vi "Man_Power Booking.vi"(6 "Man Power Details":T1={"Man Power"={"OP10"={"Clock No."="", "Name"=""}, "OP20"={"Clock No."="", "Name"=""}, "OP30"={"Clock No."="", "Name"=""}, "OP40"={"Clock No."="", "Name"=""}, "OP50"={"Clock No."="", "Name"=""}, "OP60"={"Clock No."="", "Name"=""}, "OP70"={"Clock No."="", "Name"=""}, "OP80"={"Clock No."="", "Name"=""}}, "DCODE"="", "PARTNO"="", "SERIAL NO"=28}, 8 "error in (no error)":errorcluster, 11 "Ref In":T4={"MS SQL Connection"=refnum, "UDL File"=path "", "Time"="", "DCODE"="", "WIP+1"=0, "MC No?"=0, "POKAYOKE?"=FALSE, "Expected Result"="", "Result [Status]"="", "Clock"=0.0, "RFID"="", "WIP Queue"=refnum, "TS Parameter"={"ProfitCenterCode"="", "LineCode"="", "WorkOrderNumber"="", "Model"="", "Model_with_Prefix"="", "VendorCode"="", "SetParameterDateCode"="", "PokaYoke"=0, "Target"=1, "Live_DateCode"="", "CustomerPartNumber"="", "Hand"="", "sBarcode"=FALSE, "FCA"=0, "Ent_Stamp"=timestamp(0 s since 1904-01-01), "STS_CD"=0.0}, "Data_Queue"=[], "RFID Serial No."=""} {"TS Parameter"."FCA" format="%01d"; "TS Parameter"."Target" min=1 max=100000; "TS Parameter"."PokaYoke" min=0 max=1}) -> (0 "error out":errorcluster)   [LabVIEW 2020]
uses:
  Controls/TD SQL.ctl
  <vilib>/addons/database/Connection.llb/Conn ObjectReference.ctl
  Controls/WIP_State.ctl
  Controls/TS_Parameter.ctl
  Controls/Man_Booking_Details.ctl
  Controls/Line Man Power.ctl
  Controls/Man_Power.ctl
  <userlib>/_OpenG.lib/array/array.llb/Remove Duplicates from 1D Array (String)__ogtk.vi
  <userlib>/_OpenG.lib/array/array.llb/Delete Elements from 1D Array (String)__ogtk.vi
  <vilib>/addons/database/NI_Database_API.lvlib
panel:
  out "format string":string
  out "spreadsheet string":string
  out "Man Power Booking In Progressing...":dbl(slide) scale=0.0..100.0
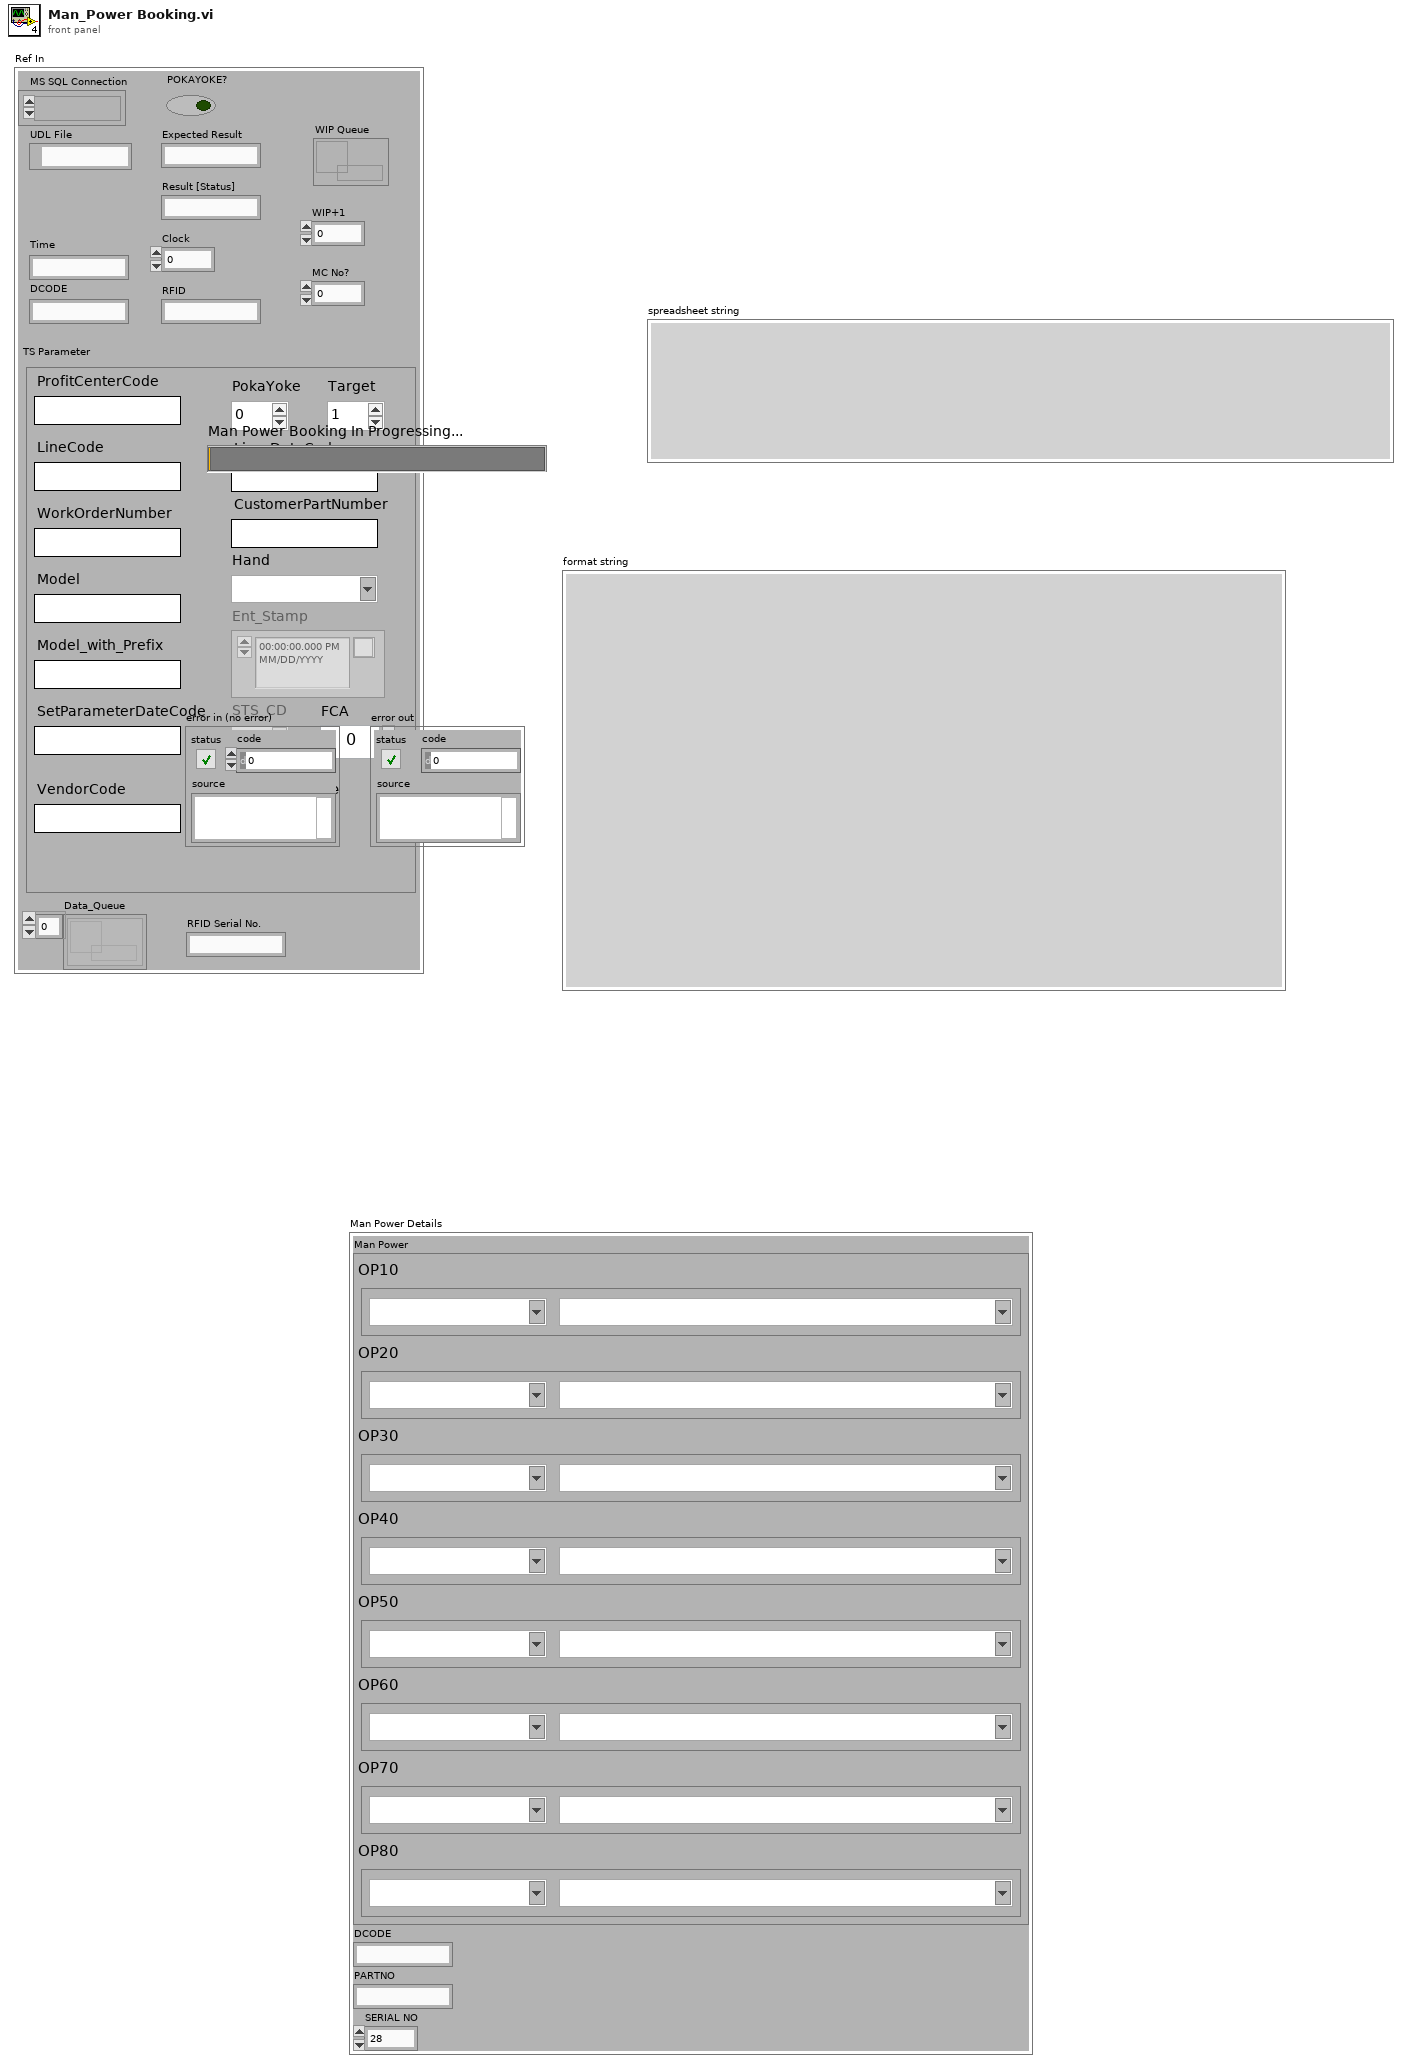
[diagram p1: front panel]
types:
  T1 = typedef "Man_Booking_Details.ctl" = cluster{"Man Power":T2, "DCODE":string, "PARTNO":string, "SERIAL NO":i32}
  T2 = typedef "Line Man Power.ctl" = cluster{"OP10":T3, "OP20":T3, "OP30":T3, "OP40":T3, "OP50":T3, "OP60":T3, "OP70":T3, "OP80":T3}
  T3 = typedef "Man_Power.ctl" = cluster{"Clock No.":string, "Name":string}
  T4 = typedef "TD SQL.ctl" = cluster{"MS SQL Connection":T5, "UDL File":path, "Time":string, "DCODE":string, "WIP+1":i64, "MC No?":i32, "POKAYOKE?":bool, "Expected Result":string, "Result [Status]":string, "Clock":dbl, "RFID":string, "WIP Queue":refnum<queue>, "TS Parameter":T6, "Data_Queue":refnum<queue>[], "RFID Serial No.":string}
  T5 = typedef "NI_Database_API.lvlib/Conn ObjectReference.ctl" = refnum<k1>
  T6 = typedef "TS_Parameter.ctl" = cluster{"ProfitCenterCode":string, "LineCode":string, "WorkOrderNumber":string, "Model":string, "Model_with_Prefix":string, "VendorCode":string, "SetParameterDateCode":string, "PokaYoke":i32, "Target":i32, "Live_DateCode":string, "CustomerPartNumber":string, "Hand":string, "sBarcode":bool, "FCA":i32, "Ent_Stamp":timestamp, "STS_CD":dbl}
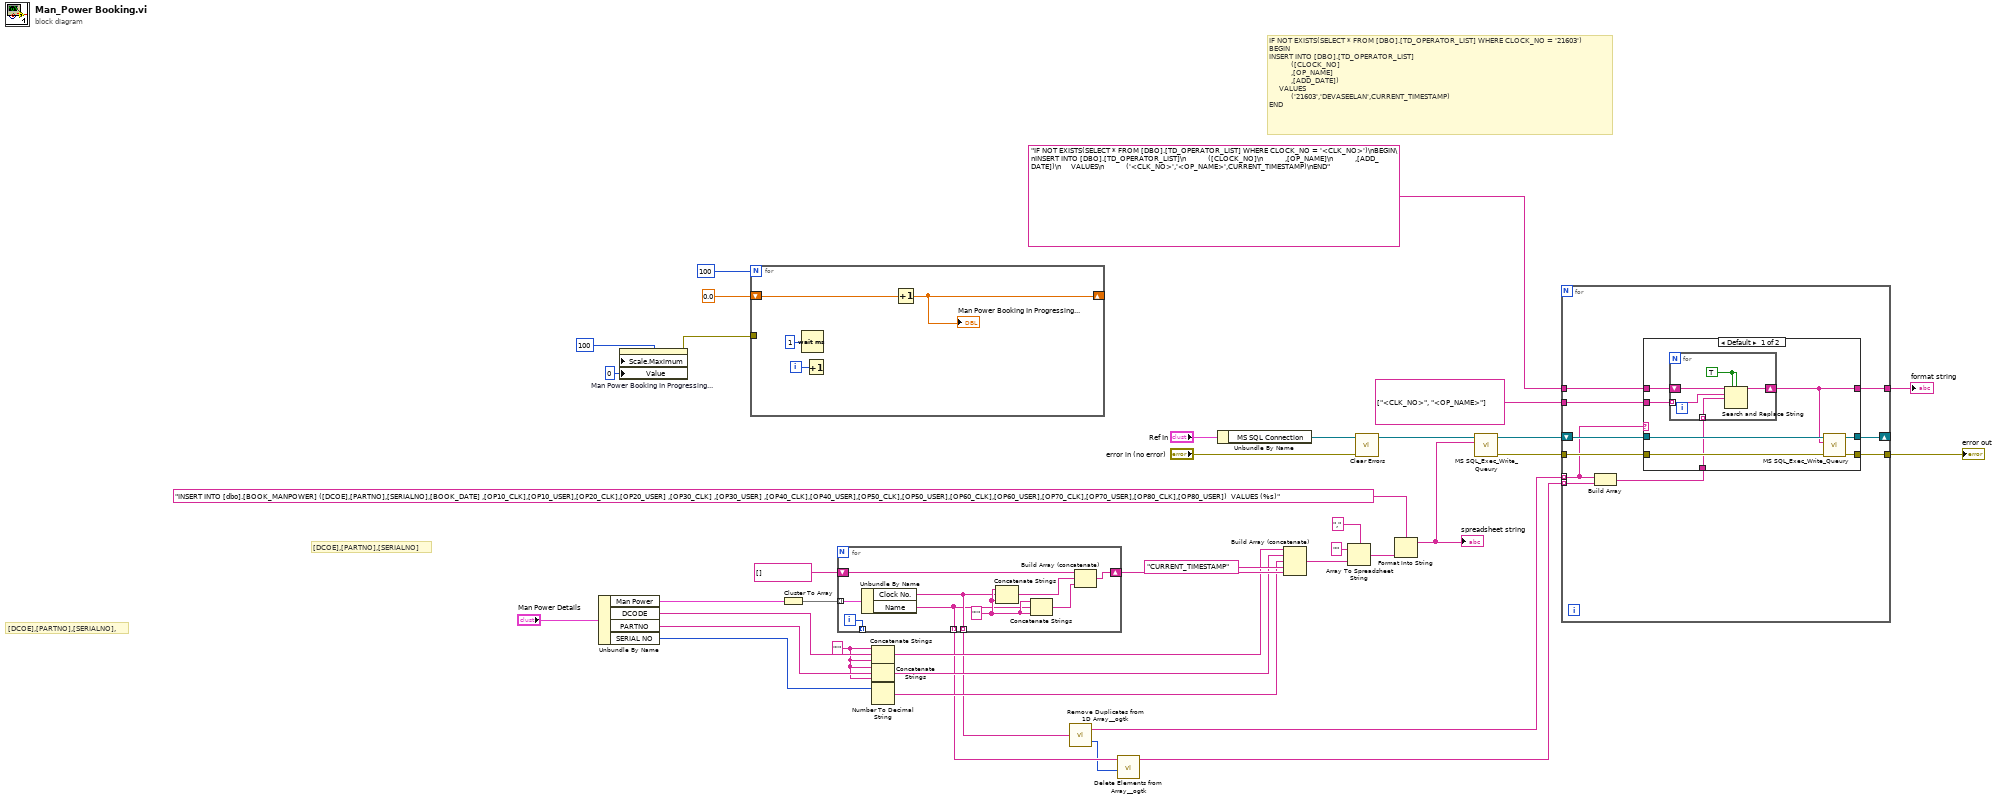
[diagram p0: block diagram]
diagram:
  w23 = "'" ("string")
  # "IF NOT EXISTS(SELECT * FROM [DBO].[TD_OPERATOR_LIST] WHERE CLOCK_NO = '21603')\nBEGIN\nINSERT INTO [DBO].[TD_OPERATOR_LIST]\n           ([CLOCK_NO]\n           ,[OP_NAME]\n           ,[ADD_DATE])\n     VALUES\n           ('21603','DEVASEELAN',CURRENT_TIMESTAMP)\nEND"
  # "[DCOE],[PARTNO],[SERIALNO]"
  # "[DCOE],[PARTNO],[SERIALNO],"
  n1 = Unbundle By Name("Man Power Details") -> ("Man Power"=w26:T2, "DCODE"=w25:string, "PARTNO"=w24:string, "SERIAL NO"=w22:i32)
  n2 = property on="Man Power Booking In Progressing..." class="Slide (strict)"("Scale.Maximum"=100 ("y"), "Value"=u8 0 ("Delete In Process...")) -> (error out=w13:errorcluster)  [unwired: 2 in, 1 out]
  n3 = for {
    N: 100 -> [_]
    shift-right: [w41] -> _
    shift-left: 0.0 ("Delete In Process...") -> [w40]
    tunnel: w13 -> [_]
    i -> [w42]
    n4 = Wait (ms)(milliseconds to wait=u32 1) -> ()  [unwired: 1 out]
    n5 = Increment(x=w42) -> ()  [unwired: 1 out]
    n6 = Increment(x=w40) -> (x+1=w41:dbl)
    "Man Power Booking In Progressing..." <- w41
  }
  n7 = Cluster To Array(cluster=w26) -> (array=w34:T3[])
  n8 = for {
    tunnel: w34 -> [w51] mode=indexing
    shift-right: [w49] -> w32
    shift-left: string[] [] -> [w50]
    tunnel: [w45] -> w11 mode=indexing
    tunnel: [w44] -> w10 mode=indexing
    tunnel: [w43] -> _ mode=indexing
    i -> [w43]
    w46 = "'" ("string")
    n9 = Unbundle By Name(w51) -> ("Clock No."=w45:string, "Name"=w44:string)
    n10 = Concatenate Strings(w46, w45, w46) -> (w48:string)
    n11 = Concatenate Strings(w46, w44, w46) -> (w47:string)
    n12 = Build Array (concatenate)(w50, w48, w47) -> (w49:string[])
  }
  n13 = Concatenate Strings(w23, w25, w23) -> (w21:string)
  n14 = Concatenate Strings(w23, w24, w23) -> (w20:string)
  n15 = Number To Decimal String(number=w22) -> (decimal integer string=w19:string)  [unwired: 1 in]
  n16 = call-poly <userlib>:"Remove Duplicates from 1D Array__ogtk.vi"("Input Array"=w11) -> ("Output Array"=w5:string[], "indices of removed elements"=w9:i32[])
  n17 = call-poly <userlib>:"Delete Elements from Array__ogtk.vi"("indices"=w9, "array"=w10) -> ("array w/ subset deleted"=w4:string[])  [unwired: 8 in, 1 out]
  n18 = Unbundle By Name("Ref In") -> ("MS SQL Connection"=w14:T5)
  n19 = Build Array (concatenate)(w21, w20, w19, "CURRENT_TIMESTAMP", w32) -> (w29:string[])
  n20 = Array To Spreadsheet String(delimiter (Tab)=",", array=w29, 3:"" ("format string")) -> (spreadsheet string=w15:string)
  n21 = call <vilib>:"Clear Errors.vi"("error in (no error)"="error in (no error)") -> ()  [unwired: 5 in, 2 out]
  n22 = Format Into String(format string="INSERT INTO [dbo].[BOOK_MANPOWER] ([DCOE],[PARTNO],[SERIALNO],[BOOK_DATE] ,[OP10_CLK],[OP10_USER],[OP20_CLK],[OP20_USER] ,[OP30_CLK] ,[OP30_USER] ,[OP40_CLK],[OP40_USER],[OP50_CLK],[OP50_USER],[OP60_CLK],[OP60_USER],[OP70_CLK],[OP70_USER],[OP80_CLK],[OP80_USER])  VALUES (%s)" ("SQL query"), w15) -> (resulting string=w12:string)  [unwired: 2 in, 1 out]
  "spreadsheet string" <- w12
  n23 = call "MS SQL_Exec_Write_Queury.vi"("Query"=w12, "Refnum in"=w14) -> ("error out"=w7:errorcluster, "Refnum out"=w8:T5)  [unwired: 8 in]
  n24 = for {
    shift-right: [w55] -> _
    shift-left: w8 -> [w61]
    tunnel: w7 -> [w60]
    tunnel: "IF NOT EXISTS(SELECT * FROM [DBO].[TD_OPERATOR_LIST] WHERE CLOCK_NO = '<CLK_NO>')\nBEGIN\nINSERT INTO [DBO].[TD_OPERATOR_LIST]\n           ([CLOCK_NO]\n           ,[OP_NAME]\n           ,[ADD_DATE])\n     VALUES\n           ('<CLK_NO>','<OP_NAME>',CURRENT_TIMESTAMP)\nEND" ("format string") -> [w58]
    tunnel: w5 -> [w52] mode=indexing
    tunnel: w4 -> [w57] mode=indexing
    tunnel: string[] ["<CLK_NO>", "<OP_NAME>"] ("array w/ subset deleted") -> [w59]
    tunnel: [w54] -> w2
    tunnel: [w53] -> w1
    n25 = Build Array(w52, w57) -> (w56:string[])
    n26 = case shown="Default" w52 {
      tunnel: w61 -> [w69 w76]
      tunnel: w60 -> [w68 w75]
      tunnel: w59 -> [w67 _]
      tunnel: w58 -> [w66 w77]
      tunnel: w56 -> [w65 _]
      tunnel: [w64 w76] -> w55
      tunnel: [w63 w75] -> w54
      tunnel: [w62 w77] -> w53
      frame Default {
        n27 = for {
          tunnel: w67 -> [w71] mode=indexing
          shift-right: [w73] -> w62
          shift-left: w66 -> [w74]
          tunnel: w65 -> [w70] mode=indexing
          w72 = TRUE ("replace all? (F)")
          n28 = Search and Replace String(replace all?=w72, case sensitive?=w72, input string=w74, search string=w71, replace string=w70) -> (result string=w73:string)  [unwired: 3 in, 3 out]
        }
        n29 = call "MS SQL_Exec_Write_Queury.vi"("error in (no error)"=w68, "Query"=w62, "Refnum in"=w69) -> ("error out"=w63:errorcluster, "Refnum out"=w64:T5)  [unwired: 7 in]
      }
      frame "" {
      }
    }
  }
  "error out" <- w2
  "format string" <- w1
